vi "X-Light V2 Device Engine.vi"(0 "XLight Notifier Name":string="XLight", 11 "COM Port":string[](array[string])) -> ()   [LabVIEW 2020]
uses:
  X-Light V2 Type Defs/X-Light Notifer Data.ctl
  X-Light V2 Type Defs/X-Light V2 Actions.ctl
  <vilib>/Instr/_visa.llb/VISA Configure Serial Port (Instr).vi
panel:
  in  "Home All":bool
  in  "Get All Positions":bool
  in  "Disk On":bool
  in  "Disk Position":i32 min=0 max=2
  in  "Dichroic":i32=1 min=1 max=5
  in  "Filter Wheel":i32=1 min=1 max=8
  out "Latest Error":errorcluster
  in  "Quit":bool
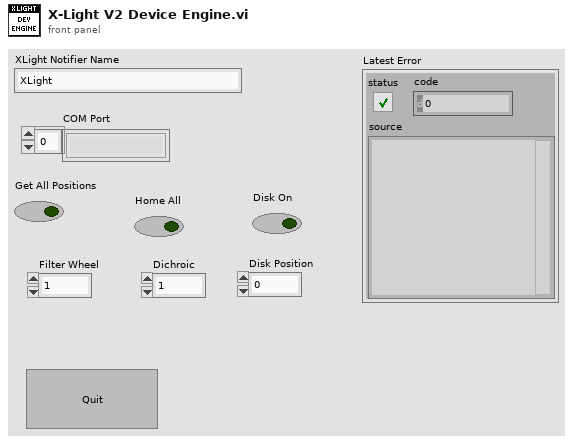
[diagram p1: front panel]
types:
  T1 = typedef "X-Light Notifer Data.ctl" = cluster{"Actions":T2, "Disk On?":bool, "Dichroic Pos.":i32, "Filter Wheel Pos.":i32, "Disk Pos.":i32, "Recived":bool}
  T2 = typedef "X-Light V2 Actions.ctl" = enum16{"Status", "Get All Pos.", "Home All", "Set Filter Wheel Pos.", "Set Disk Pos.", "Set Dichroic Pos.", "Disk On", "Disk Off", "Quit"}
  T3 = enum32{"Invalid", "Standard", "Closed", "Hidden", "Minimized", "Maximized"}
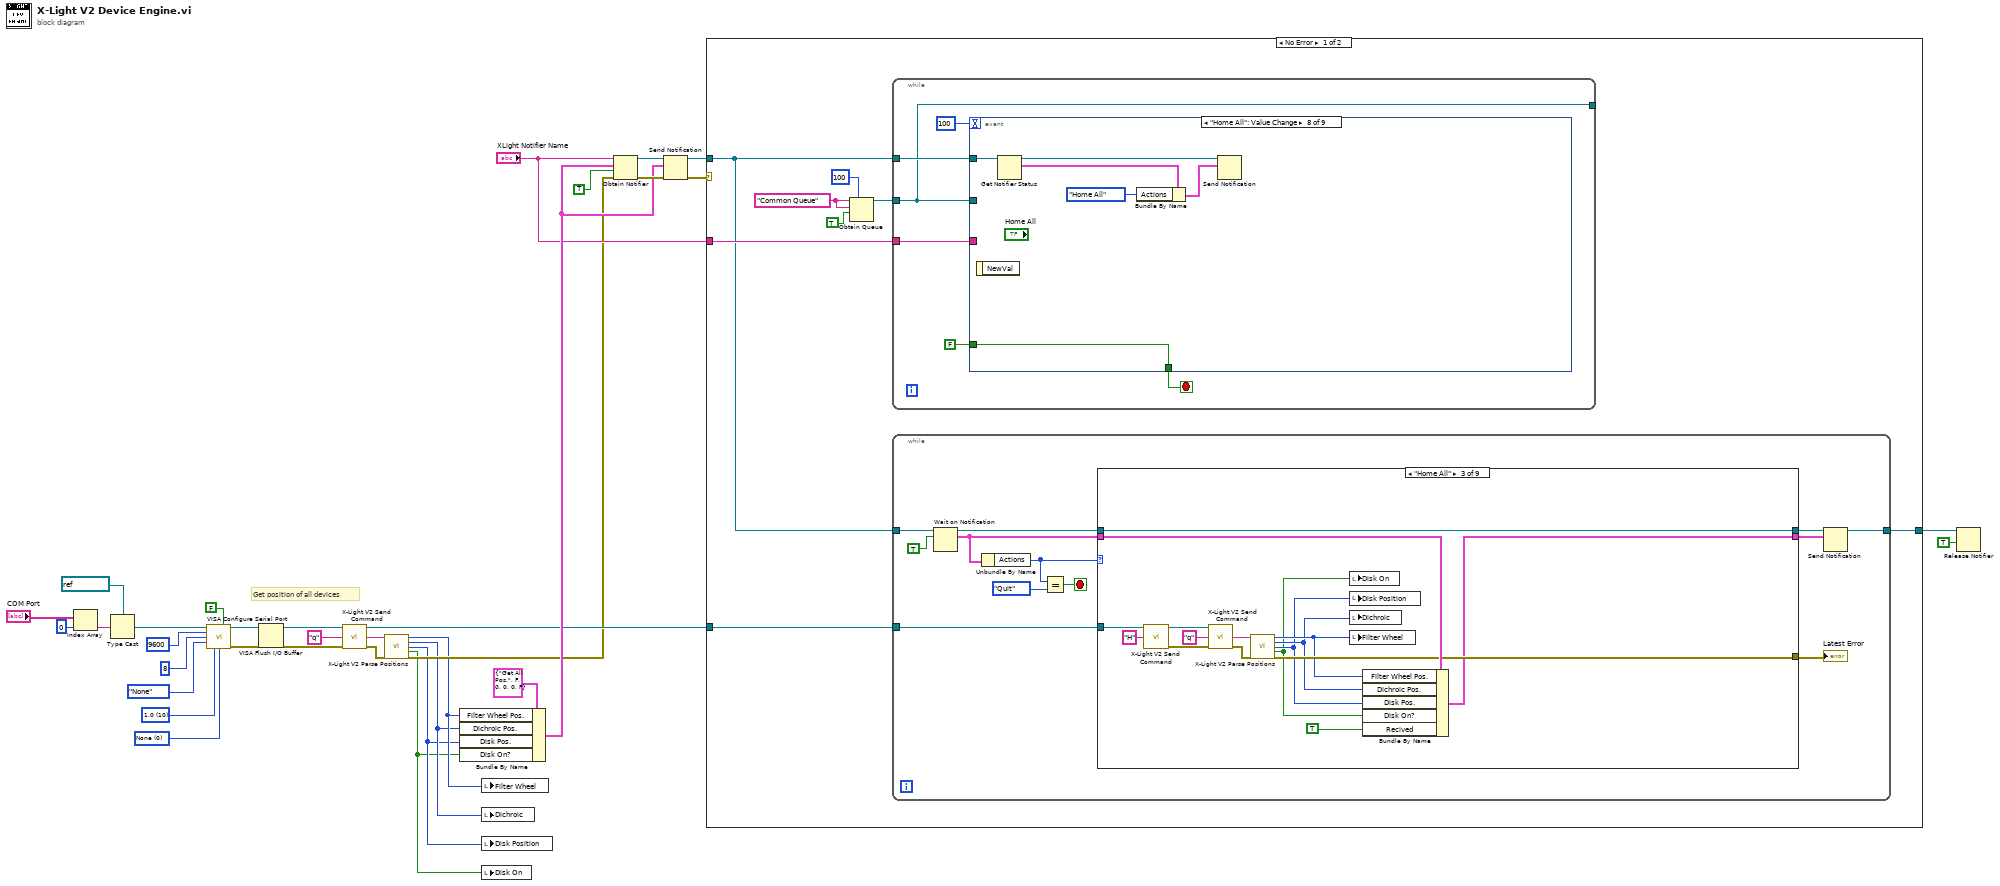
[diagram p0: block diagram]
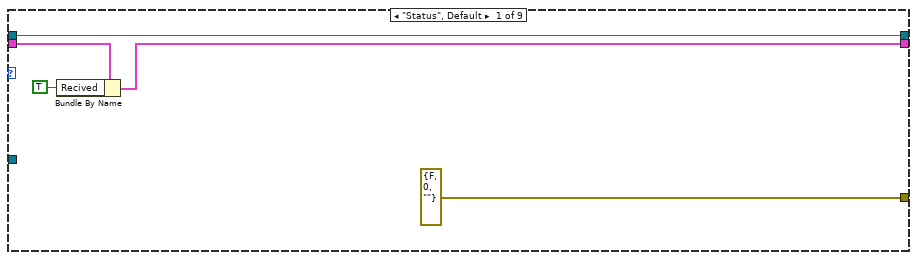
[diagram p2: hidden frame]
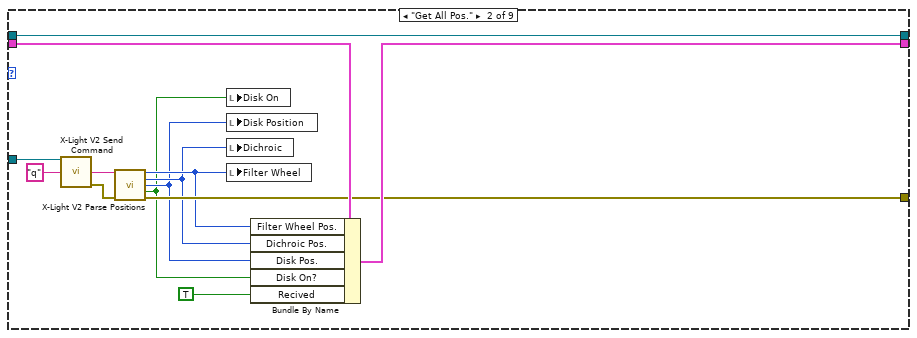
[diagram p3: hidden frame]
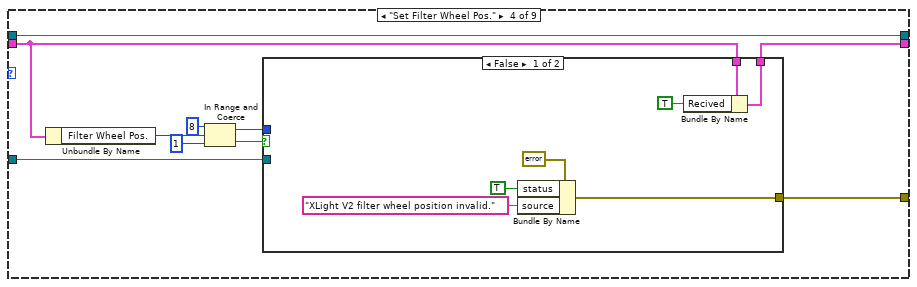
[diagram p4: hidden frame]
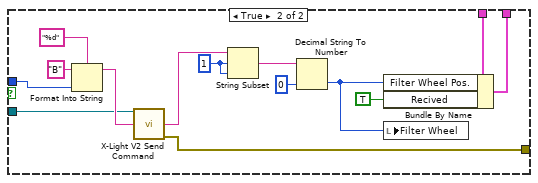
[diagram p5: hidden frame]
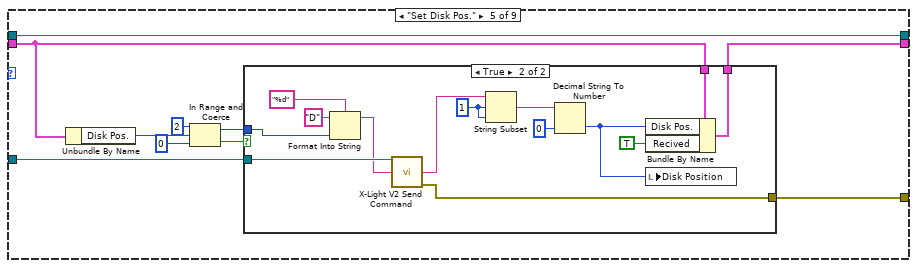
[diagram p6: hidden frame]
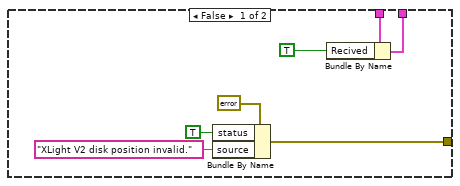
[diagram p7: hidden frame]
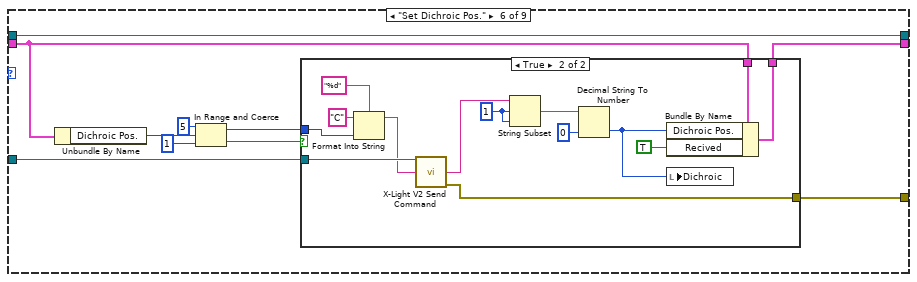
[diagram p8: hidden frame]
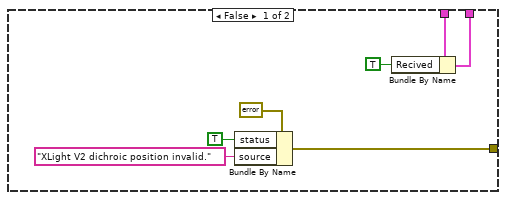
[diagram p9: hidden frame]
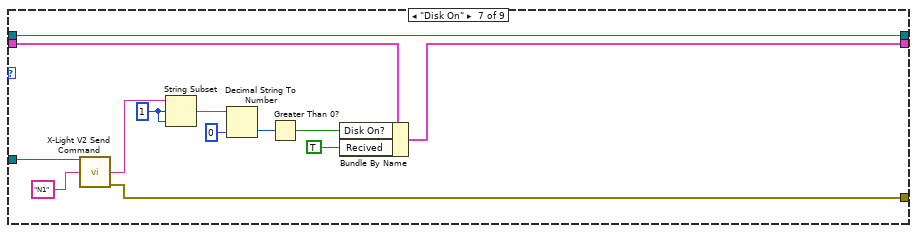
[diagram p10: hidden frame]
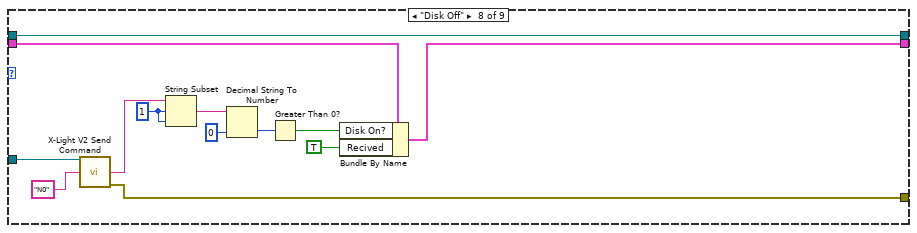
[diagram p11: hidden frame]
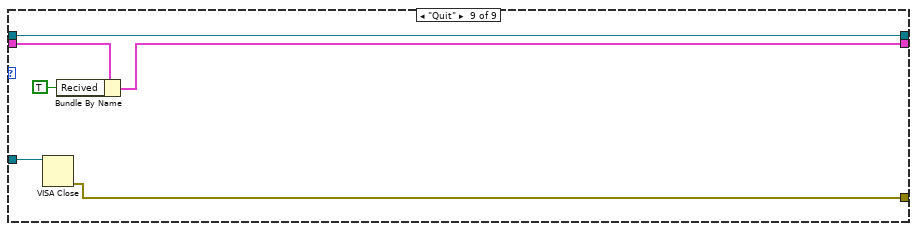
[diagram p12: hidden frame]
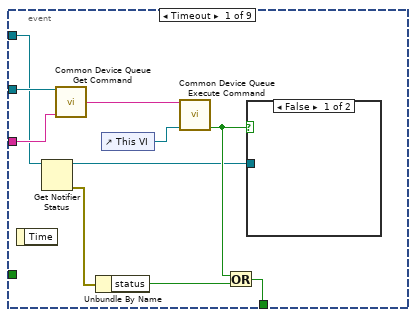
[diagram p13: hidden frame]
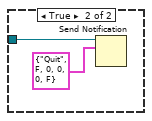
[diagram p14: hidden frame]
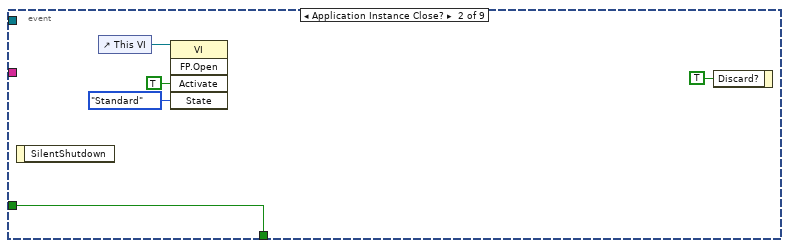
[diagram p15: hidden frame]
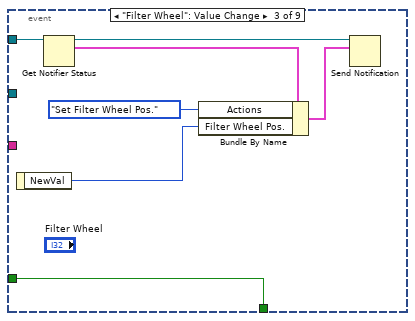
[diagram p16: hidden frame]
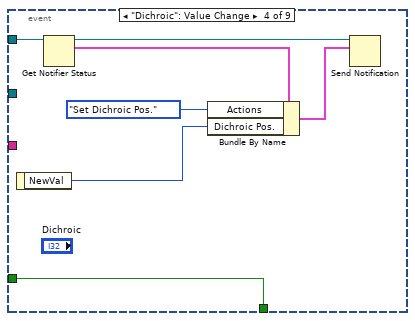
[diagram p17: hidden frame]
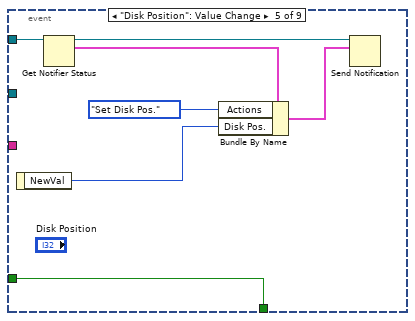
[diagram p18: hidden frame]
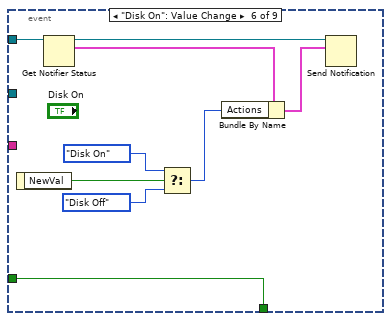
[diagram p19: hidden frame]
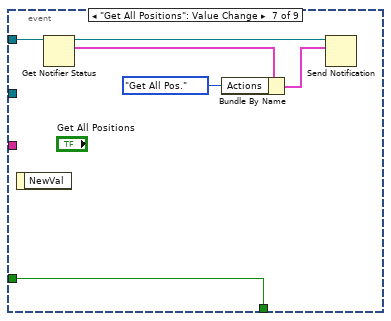
[diagram p20: hidden frame]
diagram:
  w29 = u16 0 items=["None", "XON/XOFF", "RTS/CTS", "XON/XOFF & RTS/CTS", "DTR/DSR", "XON/XOFF & DTR/DSR"] ("flow control (0:none)")
  w30 = u16 10 items=["1.0"=10, "1.5"=15, "2.0"=20] ("stop bits (10: 1 bit)")
  # "Get position of all devices"
  n1 = Index Array(array="COM Port", index=0) -> (element=w23:string)
  n2 = Type Cast(type=refnum<visa-resource-name> "COM5" ("VISA resource name"), x=w23) -> (*(type *) &x=w22:refnum<visa-resource-name>)
  n3 = call-poly "VISA Configure Serial Port"("VISA resource name"=w22, "Enable Termination\nChar (T)"=FALSE ("Enable Termination\nChar (T)"), "baud rate (9600)"=u32 9600, "data bits (8)"=u16 8, "parity (0:none)"=enum16{"None", "Odd", "Even", "Mark", "Space"}."None", "stop bits (10: 1 bit)"=w30, "flow control (0:none)"=w29) -> ("VISA resource name out"=w28:refnum<visa-resource-name>, "error out"=w27:errorcluster)  [unwired: 7 in]
  n4 = VISA Flush I/O Buffer(VISA resource name=w28, error in (no error)=w27) -> (VISA resource name out=w18:refnum<visa-resource-name>, error out=w17:errorcluster)  [unwired: 1 in]
  n5 = call "X-Light V2 Send Command.vi"("VISA Resource"=w18, "Command"="q", "Error In"=w17) -> ("VISA Resource Out"=w9:refnum<visa-resource-name>, "Reply"=w10:string, "Error Out"=w8:errorcluster)  [unwired: 10 in]
  n6 = call "X-Light V2 Parse Positions.vi"("Recived Reply"=w10, "Error In"=w8) -> ("Filter Wheel"=w4:i32, "Dichroic"=w3:i32, "Disk"=w2:i32, "Disk On"=w1:bool, "Error Out"=w7:errorcluster)  [unwired: 9 in]
  n7 = Bundle By Name(cluster=T1 {"Actions"=enum."Get All Pos.", "Disk On?"=FALSE, "Dichroic Pos."=0, "Filter Wheel Pos."=0, "Disk Pos."=0, "Recived"=FALSE} ("XLight Notifier Data"), "Filter Wheel Pos."=w4, "Dichroic Pos."=w3, "Disk Pos."=w2, "Disk On?"=w1) -> (w14:T1)
  n8 = local write "Filter Wheel"(w4) -> ()
  n9 = local write "Dichroic"(w3) -> ()
  n10 = local write "Disk Position"(w2) -> ()
  n11 = local write "Disk On"(w1) -> ()
  n12 = Obtain Notifier(name (unnamed)="XLight Notifier Name", notification data type=w14, create if not found? (T)=TRUE, error in (no error)=w7) -> (notifier out=w20:refnum<notifier>, error out=w19:errorcluster)  [unwired: 1 out]
  n13 = Send Notification(notification=w14, notifier=w20, error in (no error)=w19) -> (notifier out=w12:refnum<notifier>, error out=w13:errorcluster)
  n14 = case shown="No Error" w13 {
    tunnel: w12 -> [w36 w285]
    tunnel: w9 -> [w37 _]
    tunnel: "XLight Notifier Name" -> [w42 _]
    tunnel: [w35 w285] -> w6
    frame No Error {
      w41 = "Common Queue" ("Unique Notifier Name")
      n15 = Obtain Queue(max queue size (-1, unlimited)=100, name (unnamed)=w41, element data type=w41, create if not found? (T)=TRUE) -> (queue out=w38:refnum<queue>)  [unwired: 1 in, 2 out]
      n16 = while {
        tunnel: w38 -> [w214]
        tunnel: w42 -> [w217]
        tunnel: w36 -> [w218]
        tunnel: [w214] -> _
        stop <- w216 stop-if-true
        # "ProScan 3 GUI and Common Queue Loop"
        n17 = event shown="[7] \"Home All\": Value Change" {
          selector: _ -> [_ _ _ _ _ _ _ _ _]
          dyn-events: _ -> [_ _ _ _ _ _ _ _ _]
          timeout: 100 -> [_ _ _ _ _ _ _ _ _]
          tunnel: w214 -> [w223 _ _ _ _ _ _ _ _]
          tunnel: w218 -> [w220 _ w242 w249 w256 w265 w271 w277 w283]
          tunnel: w217 -> [w222 _ _ _ _ _ _ _ _]
          tunnel: [w221 w236 w243 w250 w257 w266 w272 w278 w284] -> w216
          tunnel: FALSE -> [_ w236 w243 w250 w257 w266 w272 w278 _]
          event Timeout {
            n18 = event-data() -> ()  [unwired: 1 in, 1 out]
            n19 = Get Notifier Status(notifier=w220) -> (notifier out=w224:refnum<notifier>, error out=w229:errorcluster)  [unwired: 1 in, 3 out]
            n20 = call "Common Device Queue Get Command.vi"("Common Queue"=w223, "Notifier Name"=w222) -> ("Command"=w228:string)  [unwired: 12 in, 1 out]
            n21 = Unbundle By Name(w229) -> ("status"=w226:bool)
            n22 = control-ref of="This VI"() -> (w227:refnum<vi>)
            n23 = call "Common Device Queue Execute Command.vi"("Common Command"=w228, "VI Refnum"=w227) -> ("Quit?"=w225:bool)  [unwired: 12 in, 1 out]
            n24 = Or(x=w225, y=w226) -> (x .or. y?=w221:bool)
            n25 = case shown="False" w225 {
              tunnel: w224 -> [_ w231]
              frame False {
              }
              frame True {
                n26 = Send Notification(notification=T1 {"Actions"=enum."Quit", "Disk On?"=FALSE, "Dichroic Pos."=0, "Filter Wheel Pos."=0, "Disk Pos."=0, "Recived"=FALSE} ("XLight Notifier Data"), notifier=w231) -> ()  [unwired: 1 in, 2 out]
              }
            }
          }
          event Application Instance Close? {
            n27 = event-data() -> ()  [unwired: 1 in, 1 out]
            n28 = control-ref of="This VI"() -> (w233:refnum<vi>)
            n29 = invoke class="VI" method="FP.Open"(reference=w233, "Activate"=TRUE ("Activate?"), "State"=T3."Standard") -> ()  [unwired: 2 in, 5 out]
            n30 = event-data("Discard?"=TRUE) -> ()  [unwired: 1 in, 1 out]
          }
          event "Filter Wheel": Value Change {
            n31 = event-data() -> ("NewVal"=w238:i32)  [unwired: 1 in]
            n32 = Get Notifier Status(notifier=w242) -> (notifier out=w241:refnum<notifier>, current notification=w240:T1)  [unwired: 1 in, 3 out]
            n33 = Bundle By Name(cluster=w240, "Actions"=X-Light_V2_Actions."Set Filter Wheel Pos.", "Filter Wheel Pos."=w238) -> (w237:T1)
            n34 = Send Notification(notification=w237, notifier=w241) -> ()  [unwired: 1 in, 2 out]
          }
          event "Dichroic": Value Change {
            n35 = event-data() -> ("NewVal"=w245:i32)  [unwired: 1 in]
            n36 = Get Notifier Status(notifier=w249) -> (notifier out=w248:refnum<notifier>, current notification=w247:T1)  [unwired: 1 in, 3 out]
            n37 = Bundle By Name(cluster=w247, "Actions"=X-Light_V2_Actions."Set Dichroic Pos.", "Dichroic Pos."=w245) -> (w244:T1)
            n38 = Send Notification(notification=w244, notifier=w248) -> ()  [unwired: 1 in, 2 out]
          }
          event "Disk Position": Value Change {
            n39 = event-data() -> ("NewVal"=w252:i32)  [unwired: 1 in]
            n40 = Get Notifier Status(notifier=w256) -> (notifier out=w255:refnum<notifier>, current notification=w254:T1)  [unwired: 1 in, 3 out]
            n41 = Bundle By Name(cluster=w254, "Actions"=X-Light_V2_Actions."Set Disk Pos.", "Disk Pos."=w252) -> (w251:T1)
            n42 = Send Notification(notification=w251, notifier=w255) -> ()  [unwired: 1 in, 2 out]
          }
          event "Disk On": Value Change {
            n43 = event-data() -> ("NewVal"=w261:bool)  [unwired: 1 in]
            n44 = Get Notifier Status(notifier=w265) -> (notifier out=w264:refnum<notifier>, current notification=w263:T1)  [unwired: 1 in, 3 out]
            n45 = Select(t=X-Light_V2_Actions."Disk On" ("Actions"), s=w261, f=X-Light_V2_Actions."Disk Off" ("Actions")) -> (s? t:f=w258:T2)
            n46 = Bundle By Name(cluster=w263, "Actions"=w258) -> (w262:T1)
            n47 = Send Notification(notification=w262, notifier=w264) -> ()  [unwired: 1 in, 2 out]
          }
          event "Get All Positions": Value Change {
            n48 = event-data() -> ()  [unwired: 1 in, 1 out]
            n49 = Get Notifier Status(notifier=w271) -> (notifier out=w270:refnum<notifier>, current notification=w269:T1)  [unwired: 1 in, 3 out]
            n50 = Bundle By Name(cluster=w269, "Actions"=X-Light_V2_Actions."Get All Pos.") -> (w268:T1)
            n51 = Send Notification(notification=w268, notifier=w270) -> ()  [unwired: 1 in, 2 out]
          }
          event "Home All": Value Change {
            n52 = event-data() -> ()  [unwired: 1 in, 1 out]
            n53 = Get Notifier Status(notifier=w277) -> (notifier out=w276:refnum<notifier>, current notification=w275:T1)  [unwired: 1 in, 3 out]
            n54 = Bundle By Name(cluster=w275, "Actions"=X-Light_V2_Actions."Home All") -> (w274:T1)
            n55 = Send Notification(notification=w274, notifier=w276) -> ()  [unwired: 1 in, 2 out]
          }
          event "Quit": Value Change {
            n56 = event-data() -> ("NewVal"=w284:bool)  [unwired: 1 in]
            n57 = Get Notifier Status(notifier=w283) -> (notifier out=w280:refnum<notifier>, current notification=w282:T1)  [unwired: 1 in, 3 out]
            n58 = Bundle By Name(cluster=w282, "Actions"=X-Light_V2_Actions."Quit") -> (w279:T1)
            n59 = Send Notification(notification=w279, notifier=w280) -> ()  [unwired: 1 in, 2 out]
          }
        }
      }
      n60 = while {
        tunnel: w37 -> [w45]
        tunnel: w36 -> [w54]
        tunnel: [w43] -> w35
        stop <- w51 stop-if-true
        n61 = Wait on Notification(notifier=w54, ignore previous (F)=TRUE) -> (notifier out=w49:refnum<notifier>, notification=w48:T1)  [unwired: 2 in, 2 out]
        n62 = Unbundle By Name(w48) -> ("Actions"=w50:T2)
        n63 = Equal?(x=w50, y=X-Light_V2_Actions."Quit") -> (x = y?=w51:bool)
        n64 = case shown="\"Home All\"" w50 {
          tunnel: w49 -> [w59 w68 w77 w98 w129 w160 w194 w207 w213]
          tunnel: w48 -> [w58 w67 w81 w96 w126 w157 w191 w204 w212]
          tunnel: [w59 w68 w77 w98 w129 w160 w194 w207 w213] -> w47
          tunnel: [w56 w65 w78 w95 w125 w156 w185 w198 w210] -> w46
          tunnel: w45 -> [_ w69 w88 w91 w128 w159 w193 w206 w209]
          tunnel: [errorcluster {"status"=FALSE, "code"=0, "source"=""} ("Error Out") w64 w79 w97 w127 w158 w192 w205 w208] -> w44
          frame "Status", Default {
            n65 = Bundle By Name(cluster=w58, "Recived"=TRUE) -> (w56:T1)
          }
          frame "Get All Pos." {
            n66 = call "X-Light V2 Send Command.vi"("VISA Resource"=w69, "Command"="q") -> ("Reply"=w71:string, "Error Out"=w70:errorcluster)  [unwired: 11 in, 1 out]
            n67 = call "X-Light V2 Parse Positions.vi"("Recived Reply"=w71, "Error In"=w70) -> ("Filter Wheel"=w63:i32, "Dichroic"=w62:i32, "Disk"=w61:i32, "Disk On"=w60:bool, "Error Out"=w64:errorcluster)  [unwired: 9 in]
            n68 = local write "Disk On"(w60) -> ()
            n69 = local write "Disk Position"(w61) -> ()
            n70 = local write "Dichroic"(w62) -> ()
            n71 = local write "Filter Wheel"(w63) -> ()
            n72 = Bundle By Name(cluster=w67, "Filter Wheel Pos."=w63, "Dichroic Pos."=w62, "Disk Pos."=w61, "Disk On?"=w60, "Recived"=TRUE) -> (w65:T1)
          }
          frame "Home All" {
            n73 = call "X-Light V2 Send Command.vi"("VISA Resource"=w88, "Command"="H") -> ("VISA Resource Out"=w83:refnum<visa-resource-name>, "Error Out"=w82:errorcluster)  [unwired: 11 in, 1 out]
            n74 = call "X-Light V2 Send Command.vi"("VISA Resource"=w83, "Command"="q", "Error In"=w82) -> ("Reply"=w85:string, "Error Out"=w84:errorcluster)  [unwired: 10 in, 1 out]
            n75 = call "X-Light V2 Parse Positions.vi"("Recived Reply"=w85, "Error In"=w84) -> ("Filter Wheel"=w76:i32, "Dichroic"=w75:i32, "Disk"=w74:i32, "Disk On"=w73:bool, "Error Out"=w79:errorcluster)  [unwired: 9 in]
            n76 = local write "Disk On"(w73) -> ()
            n77 = local write "Disk Position"(w74) -> ()
            n78 = local write "Dichroic"(w75) -> ()
            n79 = local write "Filter Wheel"(w76) -> ()
            n80 = Bundle By Name(cluster=w81, "Filter Wheel Pos."=w76, "Dichroic Pos."=w75, "Disk Pos."=w74, "Disk On?"=w73, "Recived"=TRUE) -> (w78:T1)
          }
          frame "Set Filter Wheel Pos." {
            n81 = Unbundle By Name(w96) -> ("Filter Wheel Pos."=w92:i32)
            n82 = In Range and Coerce(upper limit=8, x=w92, lower limit=1) -> (coerced(x)=w89:i32, In Range?=w90:bool)
            n83 = case shown="False" w90 {
              tunnel: [w102 w119] -> w97
              tunnel: w96 -> [w100 w115]
              tunnel: [w99 w109] -> w95
              tunnel: w91 -> [_ w108]
              tunnel: w89 -> [_ w107]
              frame False {
                n84 = Bundle By Name(cluster=errorcluster {"status"=FALSE, "code"=0, "source"=""} ("Error Out"), "status"=TRUE, "source"="XLight V2 filter wheel position invalid.") -> (w102:errorcluster)
                n85 = Bundle By Name(cluster=w100, "Recived"=TRUE) -> (w99:T1)
              }
              frame True {
                w112 = 1 ("offset (0)")
                n86 = Format Into String(format string="%d", initial string="B", w107) -> (resulting string=w116:string)  [unwired: 1 in, 1 out]
                n87 = call "X-Light V2 Send Command.vi"("VISA Resource"=w108, "Command"=w116) -> ("Reply"=w113:string, "Error Out"=w119:errorcluster)  [unwired: 11 in, 1 out]
                n88 = String Subset(string=w113, offset (0)=w112, length (rest)=w112) -> (substring=w111:string)
                n89 = Decimal String To Number(string=w111, default (0L)=0 ("default (0 I32)")) -> (number=w106:i32)  [unwired: 1 in, 1 out]
                n90 = Bundle By Name(cluster=w115, "Filter Wheel Pos."=w106, "Recived"=TRUE) -> (w109:T1)
                n91 = local write "Filter Wheel"(w106) -> ()
              }
            }
          }
          frame "Set Disk Pos." {
            n92 = Unbundle By Name(w126) -> ("Disk Pos."=w124:i32)
            n93 = In Range and Coerce(upper limit=2, x=w124, lower limit=0) -> (coerced(x)=w120:i32, In Range?=w121:bool)
            n94 = case shown="True" w121 {
              tunnel: w128 -> [_ w150]
              tunnel: [w130 w149] -> w127
              tunnel: w126 -> [w135 w145]
              tunnel: [w134 w139] -> w125
              tunnel: w120 -> [_ w138]
              frame False {
                n95 = Bundle By Name(cluster=errorcluster {"status"=FALSE, "code"=0, "source"=""} ("Error Out"), "status"=TRUE, "source"="XLight V2 disk position invalid.") -> (w130:errorcluster)
                n96 = Bundle By Name(cluster=w135, "Recived"=TRUE) -> (w134:T1)
              }
              frame True {
                w142 = 1 ("offset (0)")
                n97 = Format Into String(format string="%d", initial string="D", w138) -> (resulting string=w146:string)  [unwired: 1 in, 1 out]
                n98 = call "X-Light V2 Send Command.vi"("VISA Resource"=w150, "Command"=w146) -> ("Reply"=w143:string, "Error Out"=w149:errorcluster)  [unwired: 11 in, 1 out]
                n99 = String Subset(string=w143, offset (0)=w142, length (rest)=w142) -> (substring=w141:string)
                n100 = Decimal String To Number(string=w141, default (0L)=0 ("default (0 I32)")) -> (number=w137:i32)  [unwired: 1 in, 1 out]
                n101 = Bundle By Name(cluster=w145, "Disk Pos."=w137, "Recived"=TRUE) -> (w139:T1)
                n102 = local write "Disk Position"(w137) -> ()
              }
            }
          }
          frame "Set Dichroic Pos." {
            n103 = Unbundle By Name(w157) -> ("Dichroic Pos."=w155:i32)
            n104 = In Range and Coerce(upper limit=5, x=w155, lower limit=1) -> (coerced(x)=w153:i32, In Range?=w154:bool)
            n105 = case shown="True" w154 {
              tunnel: w159 -> [_ w181]
              tunnel: [w164 w180] -> w158
              tunnel: w153 -> [_ w179]
              tunnel: w157 -> [w162 w175]
              tunnel: [w161 w169] -> w156
              frame False {
                n106 = Bundle By Name(cluster=errorcluster {"status"=FALSE, "code"=0, "source"=""} ("Error Out"), "status"=TRUE, "source"="XLight V2 dichroic position invalid.") -> (w164:errorcluster)
                n107 = Bundle By Name(cluster=w162, "Recived"=TRUE) -> (w161:T1)
              }
              frame True {
                w172 = 1 ("offset (0)")
                n108 = Format Into String(format string="%d", initial string="C", w179) -> (resulting string=w176:string)  [unwired: 1 in, 1 out]
                n109 = call "X-Light V2 Send Command.vi"("VISA Resource"=w181, "Command"=w176) -> ("Reply"=w173:string, "Error Out"=w180:errorcluster)  [unwired: 11 in, 1 out]
                n110 = String Subset(string=w173, offset (0)=w172, length (rest)=w172) -> (substring=w171:string)
                n111 = Decimal String To Number(string=w171, default (0L)=0 ("default (0 I32)")) -> (number=w168:i32)  [unwired: 1 in, 1 out]
                n112 = Bundle By Name(cluster=w175, "Dichroic Pos."=w168, "Recived"=TRUE) -> (w169:T1)
                n113 = local write "Dichroic"(w168) -> ()
              }
            }
          }
          frame "Disk On" {
            w188 = 1 ("offset (0)")
            n114 = call "X-Light V2 Send Command.vi"("VISA Resource"=w193, "Command"="N1" ("initial string")) -> ("Reply"=w189:string, "Error Out"=w192:errorcluster)  [unwired: 11 in, 1 out]
            n115 = String Subset(string=w189, offset (0)=w188, length (rest)=w188) -> (substring=w187:string)
            n116 = Decimal String To Number(string=w187, default (0L)=0 ("default (0 I32)")) -> (number=w184:i32)  [unwired: 1 in, 1 out]
            n117 = Greater Than 0?(x=w184) -> (x > 0?=w183:bool)
            n118 = Bundle By Name(cluster=w191, "Disk On?"=w183, "Recived"=TRUE) -> (w185:T1)
          }
          frame "Disk Off" {
            w201 = 1 ("offset (0)")
            n119 = call "X-Light V2 Send Command.vi"("VISA Resource"=w206, "Command"="N0" ("initial string")) -> ("Reply"=w202:string, "Error Out"=w205:errorcluster)  [unwired: 11 in, 1 out]
            n120 = String Subset(string=w202, offset (0)=w201, length (rest)=w201) -> (substring=w200:string)
            n121 = Decimal String To Number(string=w200, default (0L)=0 ("default (0 I32)")) -> (number=w197:i32)  [unwired: 1 in, 1 out]
            n122 = Greater Than 0?(x=w197) -> (x > 0?=w196:bool)
            n123 = Bundle By Name(cluster=w204, "Disk On?"=w196, "Recived"=TRUE) -> (w198:T1)
          }
          frame "Quit" {
            n124 = VISA Close(VISA resource name=w209) -> (error out=w208:errorcluster)  [unwired: 1 in]
            n125 = Bundle By Name(cluster=w212, "Recived"=TRUE) -> (w210:T1)
          }
        }
        "Latest Error" <- w44
        n126 = Send Notification(notification=w46, notifier=w47) -> (notifier out=w43:refnum<notifier>)  [unwired: 1 in, 1 out]
      }
    }
    frame Error {
    }
  }
  n127 = Release Notifier(notifier=w6, force destroy? (F)=TRUE) -> ()  [unwired: 1 in, 3 out]
